vi "Set Direction.vi"(8 "error in (no error)":errorcluster, 10 "Direction":T1, 11 "Type Descriptor in":refnum<class "Type Descriptor.lvclass">) -> (0 "error out":errorcluster, 3 "Type Descriptor out":refnum<class "Type Descriptor.lvclass">)   [LabVIEW 2020, in "Parallel Block.lvlib" / "Type Descriptor.lvclass"]
uses:
  Type Descriptor.lvclass
  Type Descriptor.lvclass/Type Descriptor.ctl
  Direction.ctl
  Parallel Block.lvlib
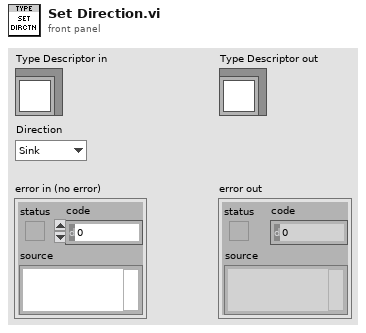
[diagram p1: front panel]
types:
  T1 = typedef "Parallel Block.lvlib/Direction.ctl" = enum16{"Sink", "Source"}
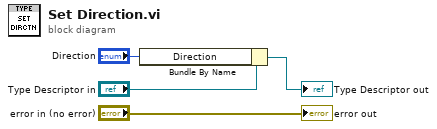
[diagram p0: block diagram]
diagram:
  n1 = Bundle By Name(cluster="Type Descriptor in", "Direction"="Direction") -> (→"Type Descriptor out":refnum<class "Type Descriptor.lvclass">)
  "error out" <- "error in (no error)"
